vi "Initialize Hardware References.vi"(4 "error in (no error)":errorcluster, 7 "Config In":T1) -> (0 "error out":errorcluster, 3 "Config Out":T1)   [LabVIEW 2019]
doc: "Initialize the hardware references."
uses:
  Settings/Settings.ctl
  Support/Hardware Configuration.ctl
  Support/Camera Configuration.ctl
  E:/DevHardSoftware/MMicroscopy/HardwareAdapter/Camera/Dependencies/PVCamNET.dll
  Camera/Dependencies/PVCamNET.dll
  <vilib>/userdefined/High Color/IMAQdx.ctl
  Logging/Logging Configuration.ctl
  controls/UI Configuration.ctl
  Global.vi
  <vilib>/vision/driver/NI_Vision_Acquisition_Software.lvlib
  Logging/Logging.lvlib
  Settings/Settings.lvlib
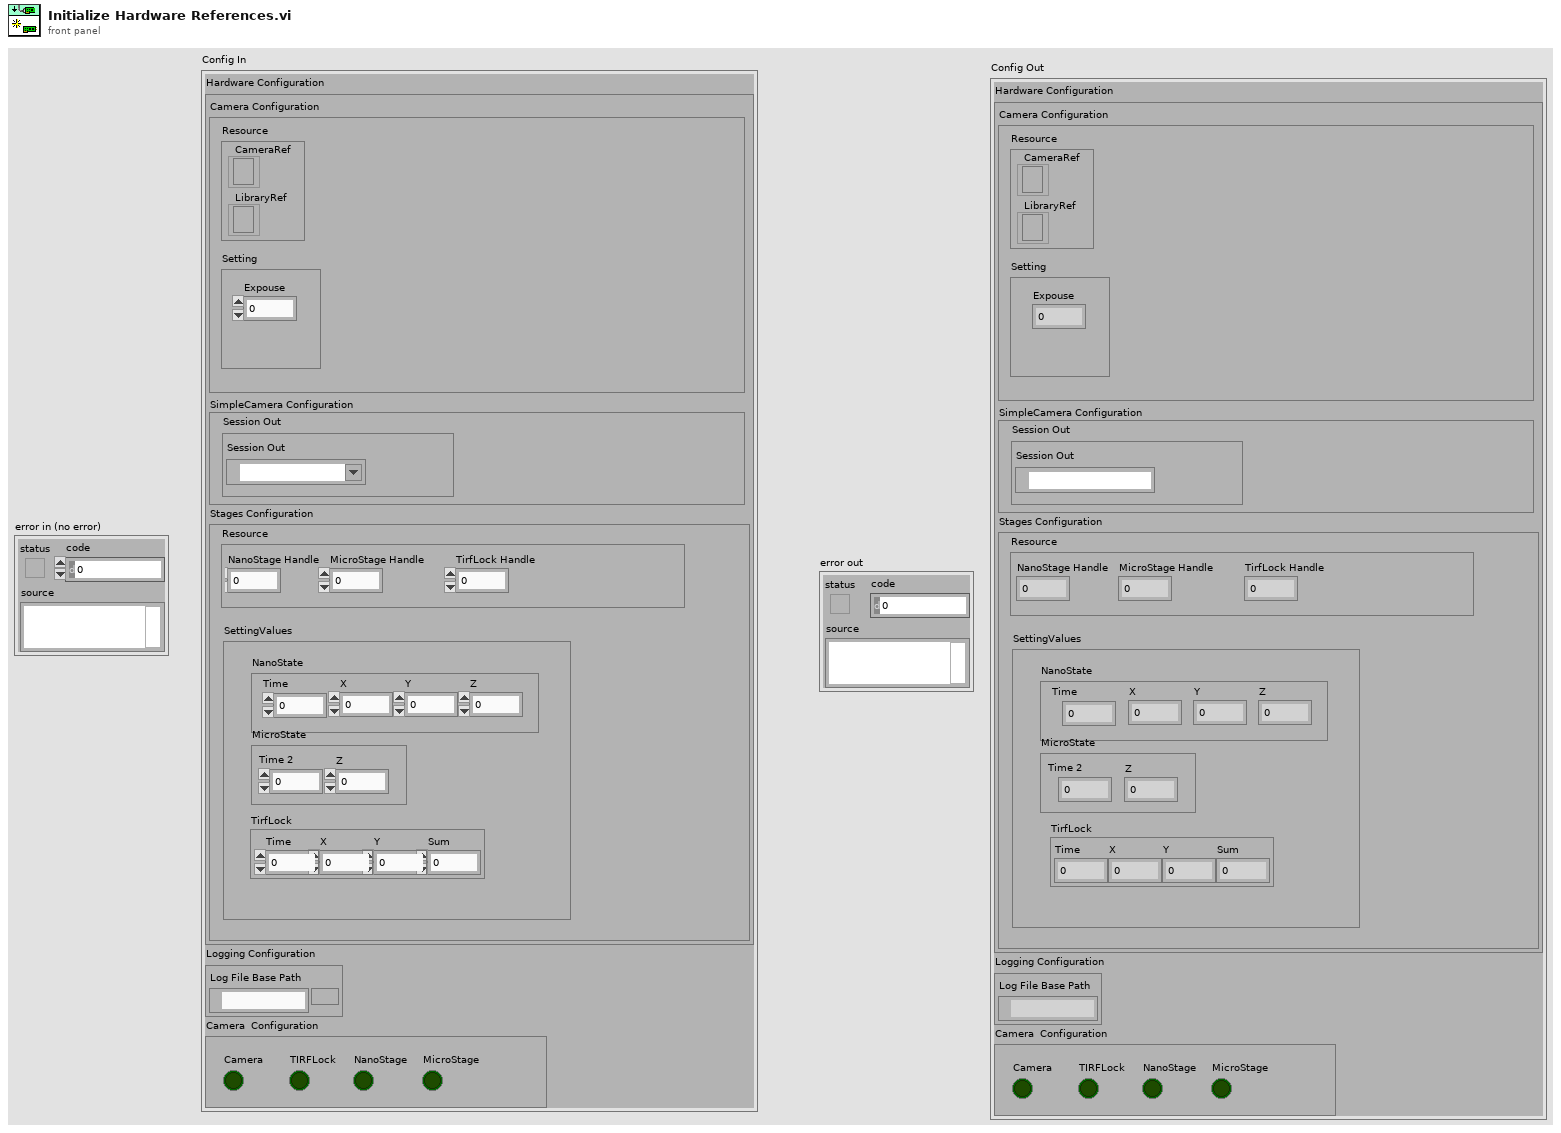
[diagram p1: front panel]
types:
  T1 = typedef "Settings.lvlib/Settings.ctl" = cluster{"Hardware Configuration":T2, "Logging Configuration":T5, "UI Configuration":T6}
  T2 = typedef "Hardware Configuration.ctl" = cluster{"Camera Configuration":T3, "SimpleCamera Configuration":cluster{"Resource":cluster{"Session Out":T4}}, "Stages Configuration":cluster{"Resource":cluster{"NanoStage Handle":i32, "MicroStage Handle":i32, "TirfLock Handle":i32}, "SettingValues":cluster{"NanoState":cluster{"Time":dbl, "X":dbl, "Y":dbl, "Z":dbl}, "MicroState":cluster{"Time 2":dbl, "Z":dbl}, "TirfLock":cluster{"Time":dbl, "X":dbl, "Y":dbl, "Sum":dbl}}}}
  T3 = typedef "Camera Configuration.ctl" = cluster{"Resource":cluster{"CameraRef":refnum<k24>, "LibraryRef":refnum<k24>}, "Setting":cluster{"Expouse":dbl}}
  T4 = typedef "IMAQdx.ctl" = refnum<k21>
  T5 = typedef "Logging.lvlib/Logging Configuration.ctl" = cluster{"Log File Base Path":path}
  T6 = typedef "UI Configuration.ctl" = cluster{"Camera":bool, "NanoStage":bool, "MicroStage":bool, "TIRFLock":bool}
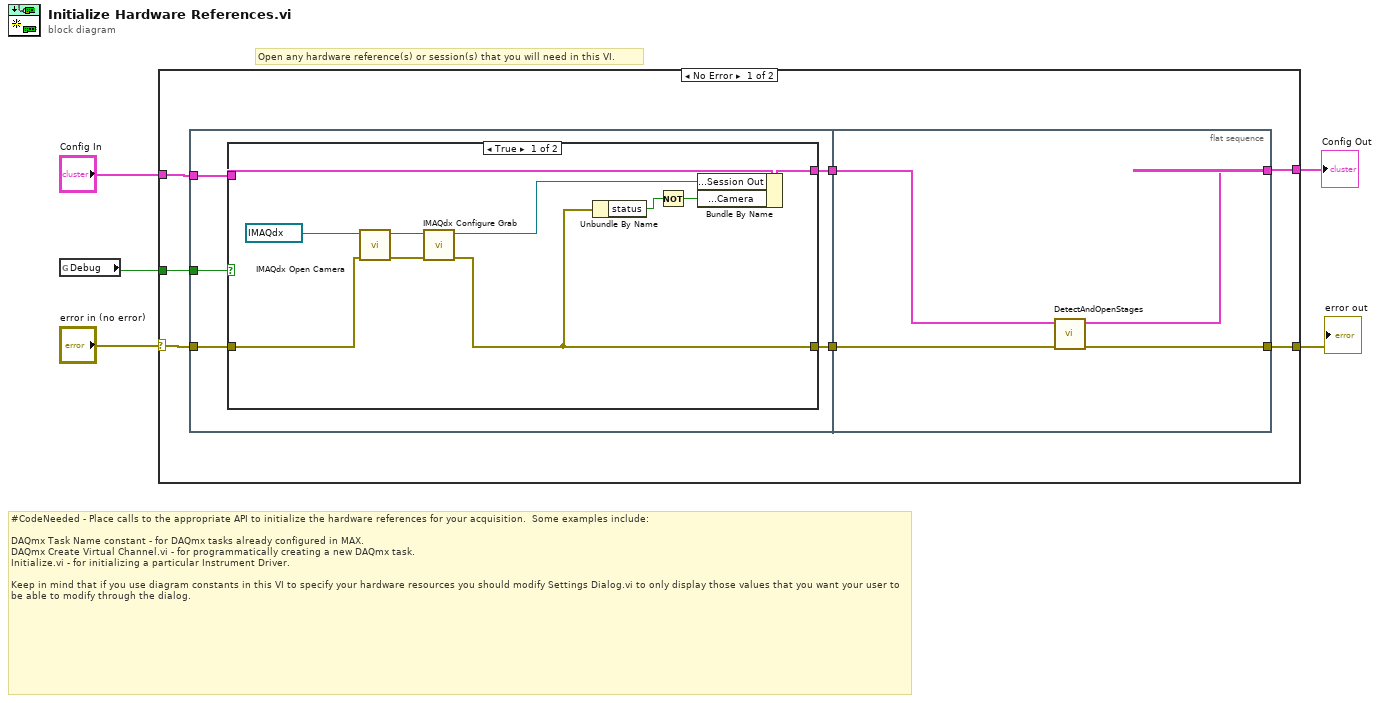
[diagram p0: block diagram]
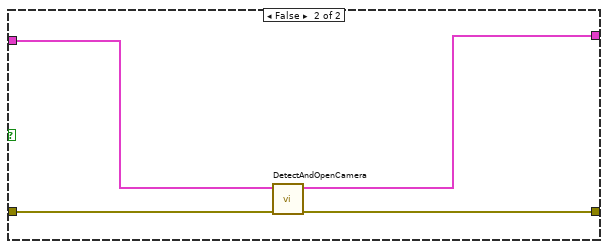
[diagram p2: hidden frame]
diagram:
  # "Open any hardware reference(s) or session(s) that you will need in this VI."
  # "#CodeNeeded - Place calls to the appropriate API to initialize the hardware references for your acquisition.  Some examples include:\n\nDAQmx Task Name constant - for DAQmx tasks already configured in MAX.\nDAQmx Create Virtual Channel.vi - for programmatically creating a new DAQmx task.\nInitialize.vi - for initializing a particular Instrument Driver.\n\nKeep in mind that if you use diagram constants in this VI to specify your hardware resources you should modify Settings Dialog.vi to only display those values that you want your user to be able to modify through the dialog."
  n1 = global read "Global.vi" "Debug"() -> (w1:bool)
  n2 = case shown="No Error" "error in (no error)" {
    selector: "error in (no error)" -> [w11 w36]
    tunnel: [w6 w36] -> w4
    tunnel: "Config In" -> [w12 w37]
    tunnel: [w10 w37] -> w2
    tunnel: w1 -> [w7 _]
    frame No Error {
      n3 = flat-sequence {
        tunnel: w12 -> [w16]
        tunnel: w11 -> [w17]
        tunnel: [w15] -> w9
        tunnel: [w14] -> w8
        tunnel: w7 -> [w13]
        tunnel: [w32] -> w10
        tunnel: w9 -> [w33]
        tunnel: w8 -> [w35]
        tunnel: [w34] -> w6
        frame #0 {
          n4 = case shown="True" w13 {
            tunnel: w17 -> [w27 w31]
            tunnel: w16 -> [w26 w29]
            tunnel: [w25 w28] -> w15
            tunnel: [w21 w30] -> w14
            frame True {
              n5 = call <vilib>:"IMAQdx Open Camera.vi"("error in"=w27, "Session In"=T4 "cam0") -> ("error out"=w18:errorcluster, "Session Out"=w19:T4)  [unwired: 8 in]
              n6 = call <vilib>:"IMAQdx Configure Grab.vi"("error in"=w18, "Session In"=w19) -> ("error out"=w21:errorcluster, "Session Out"=w24:T4)  [unwired: 8 in]
              n7 = Unbundle By Name(w21) -> ("status"=w23:bool)
              n8 = Not(x=w23) -> (.not. x?=w22:bool)
              n9 = Bundle By Name(cluster=w26, "Hardware Configuration.SimpleCamera Configuration.Resource.Session Out"=w24, "UI Configuration.Camera"=w22) -> (w25:T1)
            }
            frame False {
              n10 = call "DetectAndOpenCamera.vi"("error in (no error)"=w31, "Config In"=w29) -> ("error out"=w30:errorcluster, "Config Out"=w28:T1)  [unwired: 8 in]
            }
          }
        }
        frame #1 {
          n11 = call "DetectAndOpenStages.vi"("error in (no error)"=w35, "Config In"=w33) -> ("error out"=w34:errorcluster, "Config Out"=w32:T1)  [unwired: 8 in]
        }
      }
    }
    frame Error {
    }
  }
  "error out" <- w4
  "Config Out" <- w2
